vi "Mavlink Stop Communication.vi"(8 "error in (no error)":errorcluster, 10 "Packet Sequence In":u8, 11 "VISA in":refnum<visa-resource-name>) -> (0 "error out":errorcluster, 2 "Packet Sequence Out":u8, 3 "VISA out":refnum<visa-resource-name>)   [LabVIEW 2023]
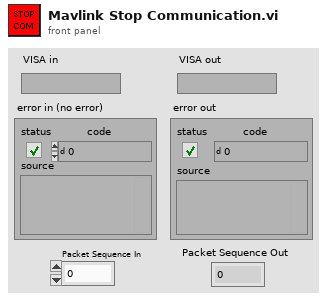
[diagram p1: front panel]
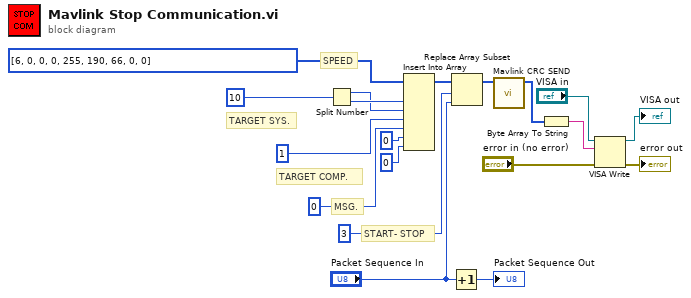
[diagram p0: block diagram]
diagram:
  # "START- STOP"
  # "TARGET COMP."
  # "TARGET SYS."
  # "SPEED"
  # "MSG."
  n1 = Split Number(x=u16 10) -> (hi(x)=w10:u8, lo(x)=w11:u8)
  n2 = Insert Into Array(array=u8[] [6, 0, 0, 0, 255, 190, 66, 0, 0] ("milliseconds to wait"), new element #1=w11, new element #2=w10, new element #3=u8 1, new element #4=u8 0, new element #5=u8 0 ("new element/subarray"), new element #6=u8 0) -> (w12:u8[])  [unwired: 1 in]
  n3 = Increment(x="Packet Sequence In") -> (x+1=→"Packet Sequence Out":u8)
  n4 = Replace Array Subset(array=w12, new element="Packet Sequence In", index=3) -> (w13:u8[])
  n5 = call "Mavlink CRC SEND.vi"("Byte In"=w13) -> ("Output Byte"=w14:u8[])  [unwired: 10 in]
  n6 = Byte Array To String(unsigned byte array=w14) -> (string=w15:string)
  n7 = VISA Write(VISA resource name="VISA in", write buffer=w15, error in (no error)="error in (no error)") -> (VISA resource name out=→"VISA out":refnum<visa-resource-name>, error out=→"error out":errorcluster)  [unwired: 1 out]
